vi "BatteryHPPCTest.vi"() -> ()   [LabVIEW 2020]
uses:
  <instrlib>/NH Research Regenerative Test Series/Public/Configure/Output Safety.ctl
  <instrlib>/NH Research Regenerative Test Series/NH Research Regenerative Test Series.lvlib
panel:
  out "error out":errorcluster
  out "Wait after discharge":dbl caption="Elapsed Time (s)"
  out "wait before discharge":dbl caption="Elapsed Time (s)"
  out "wait after pulse":dbl caption="Elapsed Time (s)"
  out "initial Wait":dbl caption="Elapsed Time (s)"
  in  "DAQmx Task Name":refnum<k21>
  out "String":string
  in  "5-SOC steps":T1 {"Voltage Setpoint (0 V) 3" format="%#.6g"; "Current Setpoint (0 A) 3" format="%#.6g"; "Power Setpoint (0 W) 3" format="%#.6g"; "Resistance Setpoint (0 Ohms) 3" format="%#.6g"; "Voltage Setpoint (0 V) 2" format="%#.6g"; "Current Setpoint (0 A) 2" format="%#.6g"; "Power Setpoint (0 W) 2" format="%#.6g"; "Resistance Setpoint (0 Ohms) 2" format="%#.6g"; "Voltage Setpoint (0 V)" format="%#.6g"; "Current Setpoint (0 A)" format="%#.6g"; "Power Setpoint (0 W)" format="%#.6g"; "Resistance Setpoint (0 Ohms)" format="%#.6g"; "Battery Detect Voltage (0V)" format="%#.6g"}
  in  "10-SOC steps":T2 {"Voltage Setpoint (0 V) 3" format="%#.6g"; "Current Setpoint (0 A) 3" format="%#.6g"; "Power Setpoint (0 W) 3" format="%#.6g"; "Resistance Setpoint (0 Ohms) 3" format="%#.6g"; "Voltage Setpoint (0 V) 2" format="%#.6g"; "Current Setpoint (0 A) 2" format="%#.6g"; "Power Setpoint (0 W) 2" format="%#.6g"; "Resistance Setpoint (0 Ohms) 2" format="%#.6g"; "Voltage Setpoint (0 V)" format="%#.6g"; "Current Setpoint (0 A)" format="%#.6g"; "Power Setpoint (0 W)" format="%#.6g"; "Resistance Setpoint (0 Ohms)" format="%#.6g"; "Battery Detect Voltage (0V)" format="%#.6g"}
  in  "#5-SOC steps":i32
  in  "#10-SOC Steps":i32
  in  "Output Safety":T3
  in  "VISA resource name":refnum<visa-resource-name>
  # "For Discharge Pulse:"
  # "For Charge Pulse:"
  # "For  5SOC discharge:"
  # "For Discharge Pulse:"
  # "For Charge Pulse:"
  # "For  10SOC discharge:"
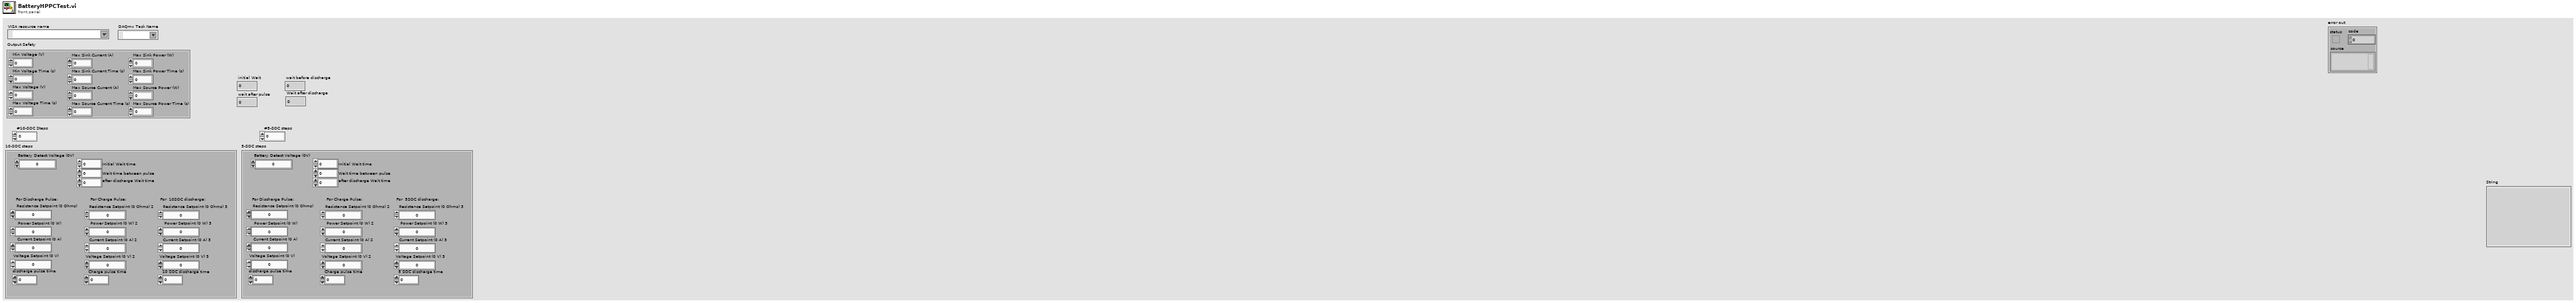
[diagram p1: front panel]
types:
  T1 = cluster{"Battery Detect Voltage (0V)":dbl, "Initial Wait time":dbl, "Resistance Setpoint (0 Ohms)":dbl, "Power Setpoint (0 W)":dbl, "Current Setpoint (0 A)":dbl, "Voltage Setpoint (0 V)":dbl, "Wait time between pulse":dbl, "after discharge Wait time ":dbl, "Resistance Setpoint (0 Ohms) 2":dbl, "Power Setpoint (0 W) 2":dbl, "Current Setpoint (0 A) 2":dbl, "Voltage Setpoint (0 V) 2":dbl, "Resistance Setpoint (0 Ohms) 3":dbl, "Power Setpoint (0 W) 3":dbl, "Current Setpoint (0 A) 3":dbl, "Voltage Setpoint (0 V) 3":dbl, "discharge pulse time":dbl, "Charge pulse time ":dbl, "5 SOC discharge time":dbl}
  T2 = cluster{"Battery Detect Voltage (0V)":dbl, "Initial Wait time":dbl, "Resistance Setpoint (0 Ohms)":dbl, "Power Setpoint (0 W)":dbl, "Current Setpoint (0 A)":dbl, "Voltage Setpoint (0 V)":dbl, "Wait time between pulse":dbl, "after discharge Wait time ":dbl, "Resistance Setpoint (0 Ohms) 2":dbl, "Power Setpoint (0 W) 2":dbl, "Current Setpoint (0 A) 2":dbl, "Voltage Setpoint (0 V) 2":dbl, "Resistance Setpoint (0 Ohms) 3":dbl, "Power Setpoint (0 W) 3":dbl, "Current Setpoint (0 A) 3":dbl, "Voltage Setpoint (0 V) 3":dbl, "discharge pulse time":dbl, "Charge pulse time ":dbl, "10 SOC discharge time":dbl}
  T3 = typedef "NH Research Regenerative Test Series.lvlib/Output Safety.ctl" = cluster{"Min Voltage (V)":dbl, "Min Voltage Time (s)":dbl, "Max Voltage (V)":dbl, "Max Voltage Time (s)":dbl, "Max Sink Current (A)":dbl, "Max Sink Current Time (s)":dbl, "Max Source Current (A)":dbl, "Max Source Current Time (s)":dbl, "Max Sink Power (W)":dbl, "Max Sink Power Time (s)":dbl, "Max Source Power (W)":dbl, "Max Source Power Time (s)":dbl}
  T4 = cluster{"[0]":refnum<visa-resource-name>, "[1]":refnum<visa-resource-name>, "[2]":refnum<visa-resource-name>, "[3]":refnum<visa-resource-name>, "[4]":refnum<visa-resource-name>, "[5]":refnum<visa-resource-name>, "[6]":refnum<visa-resource-name>, "[7]":refnum<visa-resource-name>, "[8]":refnum<visa-resource-name>}
  T5 = cluster{"[0]":refnum<k21>, "[1]":refnum<k21>, "[2]":refnum<k21>, "[3]":refnum<k21>, "[4]":refnum<k21>, "[5]":refnum<k21>, "[6]":refnum<k21>, "[7]":refnum<k21>, "[8]":refnum<k21>}
  T6 = cluster{"[0]":errorcluster, "[1]":errorcluster, "[2]":errorcluster, "[3]":errorcluster, "[4]":errorcluster, "[5]":errorcluster, "[6]":errorcluster, "[7]":errorcluster, "[8]":errorcluster}
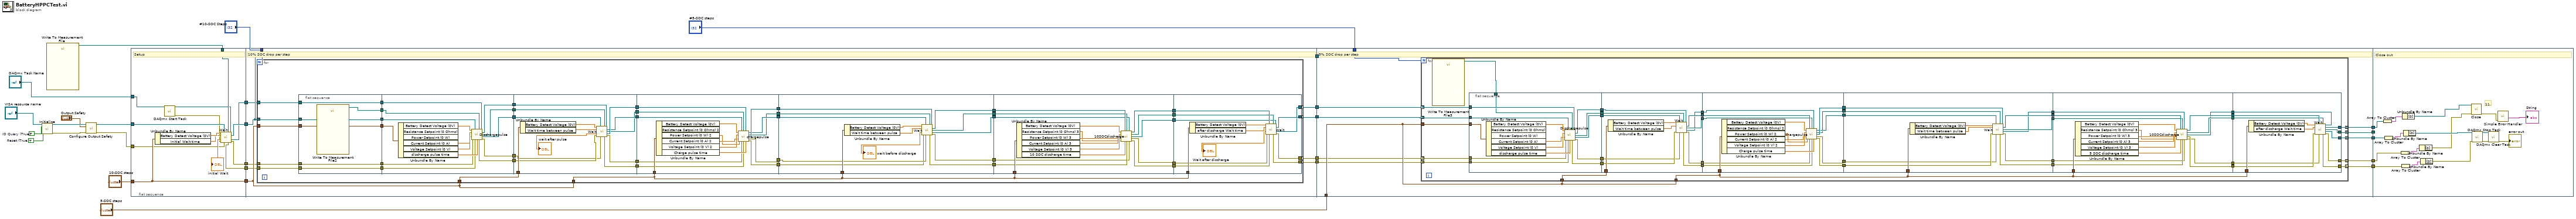
[diagram p0: block diagram]
diagram:
  w28 = TRUE  # ID Query (True)
  w27 = TRUE  # Reset (True)
  n1 = call <vilib>:"Initialize.vi"("VISA resource name"="VISA resource name", "ID Query (True)"=w28, "Reset (True)"=w27) -> ("VISA resource name out"=w26:refnum<visa-resource-name>, "error out"=w25:errorcluster)  [unwired: 11 in]
  n2 = call "Write To Measurement File"() -> ("Filename Out"=w11:path)  [unwired: 17 in, 2 out]
  n3 = call <vilib>:"Configure Output Safety.vi"("VISA resource name"=w26, "Output Safety"="Output Safety", "error in (no error)"=w25) -> ("VISA resource name out"=w23:refnum<visa-resource-name>, "error out"=w10:errorcluster)  [unwired: 11 in]
  n4 = flat-sequence {
    tunnel: w23 -> [w35]
    tunnel: [w36] -> w20
    tunnel: "10-SOC steps" -> [w43]
    tunnel: [w43] -> w17
    tunnel: "DAQmx Task Name" -> [w30]
    tunnel: [w33] -> w14
    tunnel: w11 -> [w34]
    tunnel: w10 -> [w39]
    tunnel: [w38] -> w9
    tunnel: [w37] -> w8
    tunnel: "#10-SOC Steps" -> [w53]
    tunnel: w20 -> [w50]
    tunnel: [w52] -> w19
    tunnel: w17 -> [w51]
    tunnel: [w50] -> w15
    tunnel: w14 -> [w49]
    tunnel: [w48] -> w13
    tunnel: w9 -> [w47]
    tunnel: w8 -> [w46]
    tunnel: [w45] -> w7
    tunnel: [w44] -> w6
    tunnel: "#5-SOC steps" -> [w200]
    tunnel: w19 -> [w201]
    tunnel: "5-SOC steps" -> [w199]
    tunnel: w15 -> [_]
    tunnel: w13 -> [w198]
    tunnel: w7 -> [w197]
    tunnel: w6 -> [w196]
    tunnel: [w195] -> w5
    tunnel: [w194] -> w4
    tunnel: [w193] -> w3
    tunnel: [w192] -> w2
    tunnel: [w191] -> w1
    tunnel: w5 -> [w336]
    tunnel: w4 -> [w338]
    tunnel: w3 -> [w342]
    tunnel: w2 -> [_]
    tunnel: w1 -> [w340]
    frame #0 {
      # "Setup"
      n5 = Unbundle By Name(w43) -> ("Battery Detect Voltage (0V)"=w42:dbl, "Initial Wait time"=w41:dbl)
      n6 = call <vilib>:"DAQmx Start Task.vi"("task/channels in"=w30) -> ("task out"=w31:refnum<k21>, "error out"=w32:errorcluster)  [unwired: 13 in]
      n7 = call "Wait.vi"("Battery Detect Voltage (0V)"=w42, "VISA resource name"=w35, "Path"=w34, "DAQmx Task Name"=w31, "Wait time"=w41, "Task error in"=w32, "Visa error in (no error)"=w39) -> ("VISA resource name out"=w36:refnum<visa-resource-name>, "WaitElapsed Time (s)"=→"initial Wait":dbl, "task out"=w33:refnum<k21>, "Task error out"=w37:errorcluster, "Visa error out"=w38:errorcluster)  [unwired: 3 in, 1 out]
    }
    frame #1 {
      # "10% SOC drop per step"
      n8 = for {
        N: w53 -> [_]
        tunnel: w50 -> [w91]
        tunnel: [w90] -> w52 mode=indexing
        tunnel: w51 -> [w89]
        tunnel: w51 -> [w88]
        tunnel: w51 -> [w87]
        tunnel: w49 -> [w86]
        tunnel: [w80] -> w48 mode=indexing
        tunnel: w47 -> [w79]
        tunnel: w46 -> [w78]
        tunnel: [w61] -> w45 mode=indexing
        tunnel: [w60] -> w44 mode=indexing
        n9 = flat-sequence {
          tunnel: w78 -> [w97]
          tunnel: w79 -> [w98]
          tunnel: w86 -> [w99]
          tunnel: w89 -> [w100]
          tunnel: w91 -> [w101]
          tunnel: [w101] -> w59
          tunnel: [w100] -> w58
          tunnel: [w99] -> w57
          tunnel: [w98] -> w56
          tunnel: [w97] -> w55
          tunnel: [w96] -> w54
          tunnel: [w104] -> w95
          tunnel: [w105] -> w85
          tunnel: [w109] -> w77
          tunnel: [w108] -> w76
          tunnel: [w103] -> w75
          tunnel: w59 -> [w107]
          tunnel: w58 -> [w116]
          tunnel: w57 -> [w106]
          tunnel: w56 -> [w111]
          tunnel: w55 -> [w110]
          tunnel: w54 -> [w102]
          tunnel: w95 -> [w119]
          tunnel: [w121] -> w94
          tunnel: w88 -> [w130]
          tunnel: w85 -> [w118]
          tunnel: [w122] -> w84
          tunnel: w77 -> [w126]
          tunnel: w76 -> [w125]
          tunnel: w75 -> [w117]
          tunnel: [w124] -> w74
          tunnel: [w123] -> w73
          tunnel: [w120] -> w72
          tunnel: w94 -> [w131]
          tunnel: [w135] -> w93
          tunnel: w87 -> [w146]
          tunnel: w84 -> [w132]
          tunnel: [w136] -> w83
          tunnel: w74 -> [w139]
          tunnel: w73 -> [w140]
          tunnel: w72 -> [w133]
          tunnel: [w134] -> w71
          tunnel: [w138] -> w70
          tunnel: [w137] -> w69
          tunnel: w93 -> [w156]
          tunnel: w87 -> [w160]
          tunnel: w83 -> [w154]
          tunnel: [w152] -> w82
          tunnel: w71 -> [w155]
          tunnel: w70 -> [w149]
          tunnel: w69 -> [w150]
          tunnel: [w153] -> w68
          tunnel: [w151] -> w67
          tunnel: [w148] -> w65
          tunnel: [w147] -> w64
          tunnel: [w167] -> w92
          tunnel: w87 -> [w177]
          tunnel: w82 -> [w170]
          tunnel: [w166] -> w81
          tunnel: w68 -> [w169]
          tunnel: w67 -> [w168]
          tunnel: [w165] -> w66
          tunnel: w65 -> [w164]
          tunnel: w64 -> [w163]
          tunnel: [w162] -> w63
          tunnel: [w161] -> w62
          tunnel: w92 -> [w184]
          tunnel: [w181] -> w90
          tunnel: w87 -> [w190]
          tunnel: w81 -> [w182]
          tunnel: [w180] -> w80
          tunnel: w66 -> [w183]
          tunnel: w63 -> [w185]
          tunnel: w62 -> [w186]
          tunnel: [w179] -> w61
          tunnel: [w178] -> w60
          frame #0 {
            n10 = call "Write To Measurement File2"() -> ("Filename Out"=w96:path)  [unwired: 17 in, 2 out]
          }
          frame #1 {
            n11 = Unbundle By Name(w116) -> ("Battery Detect Voltage (0V)"=w115:dbl, "Current Setpoint (0 A)"=w113:dbl, "Voltage Setpoint (0 V)"=w114:dbl, "discharge pulse time"=w112:dbl)  [unwired: 2 out]
            n12 = call "Dischargepulse.vi"("Battery Detect Voltage (0V)"=w115, "VISA resource name"=w107, "Path"=w102, "DAQmx Task Name"=w106, "Voltage Setpoint (0 V)"=w114, "Current Setpoint (0 A)"=w113, "error in (no error)"=w111, "Task error in"=w110, "pulse time"=w112) -> ("task out"=w105:refnum<k21>, "Filename Out"=w103:path, "VISA resource name out"=w104:refnum<visa-resource-name>, "Task error out 2"=w109:errorcluster, "error out"=w108:errorcluster)  [unwired: 2 in]
          }
          frame #2 {
            n13 = Unbundle By Name(w130) -> ("Battery Detect Voltage (0V)"=w129:dbl, "Wait time between pulse"=w128:dbl)
            n14 = call "Wait.vi"("Battery Detect Voltage (0V)"=w129, "VISA resource name"=w119, "Path"=w117, "DAQmx Task Name"=w118, "Wait time"=w128, "Task error in"=w126, "Visa error in (no error)"=w125) -> ("VISA resource name out"=w121:refnum<visa-resource-name>, "Filename Out"=w120:path, "WaitElapsed Time (s)"=→"wait after pulse":dbl, "task out"=w122:refnum<k21>, "Task error out"=w124:errorcluster, "Visa error out"=w123:errorcluster)  [unwired: 3 in]
          }
          frame #3 {
            n15 = Unbundle By Name(w146) -> ("Battery Detect Voltage (0V)"=w145:dbl, "Power Setpoint (0 W) 2"=w142:dbl, "Current Setpoint (0 A) 2"=w143:dbl, "Voltage Setpoint (0 V) 2"=w144:dbl, "Charge pulse time"=w141:dbl)  [unwired: 1 out]
            n16 = call "chargepulse.vi"("Battery Detect Voltage (0V)"=w145, "VISA resource name"=w131, "Path"=w133, "DAQmx Task Name"=w132, "Voltage Setpoint (0 V)"=w144, "Current Setpoint (0 A)"=w143, "Power Setpoint (0 W)"=w142, "error in (no error)"=w140, "Task error in"=w139, "pulse time"=w141) -> ("VISA resource name out"=w135:refnum<visa-resource-name>, "Filename Out"=w134:path, "task out"=w136:refnum<k21>, "error out"=w137:errorcluster, "Task error out"=w138:errorcluster)  [unwired: 1 in]
          }
          frame #4 {
            n17 = Unbundle By Name(w160) -> ("Battery Detect Voltage (0V)"=w159:dbl, "Wait time between pulse"=w158:dbl)
            n18 = call "Wait.vi"("Battery Detect Voltage (0V)"=w159, "VISA resource name"=w156, "Path"=w155, "DAQmx Task Name"=w154, "Wait time"=w158, "Task error in"=w149, "Visa error in (no error)"=w150) -> ("VISA resource name out"=w152:refnum<visa-resource-name>, "Filename Out"=w151:path, "WaitElapsed Time (s)"=→"wait before discharge":dbl, "task out"=w153:refnum<k21>, "Task error out"=w148:errorcluster, "Visa error out"=w147:errorcluster)  [unwired: 3 in]
          }
          frame #5 {
            n19 = Unbundle By Name(w177) -> ("Battery Detect Voltage (0V)"=w176:dbl, "Resistance Setpoint (0 Ohms) 3"=w172:dbl, "Power Setpoint (0 W) 3"=w173:dbl, "Current Setpoint (0 A) 3"=w174:dbl, "Voltage Setpoint (0 V) 3"=w175:dbl, "10 SOC discharge time"=w171:dbl)
            n20 = call "10SOCdischarge.vi"("Battery Detect Voltage (0V)"=w176, "VISA resource name"=w170, "Path"=w168, "DAQmx Task Name"=w169, "Voltage Setpoint (0 V)"=w175, "Current Setpoint (0 A)"=w174, "Power Setpoint (0 W)"=w173, "Resistance Setpoint (0 Ohms)"=w172, "Discharge time"=w171, "Task error in"=w164, "error in (no error)"=w163) -> ("VISA resource name out"=w167:refnum<visa-resource-name>, "Filename Out"=w165:path, "task out"=w166:refnum<k21>, "Task error out 2"=w161:errorcluster, "error out"=w162:errorcluster)
          }
          frame #6 {
            n21 = Unbundle By Name(w190) -> ("Battery Detect Voltage (0V)"=w189:dbl, "after discharge Wait time"=w188:dbl)
            n22 = call "Wait.vi"("Battery Detect Voltage (0V)"=w189, "VISA resource name"=w184, "Path"=w183, "DAQmx Task Name"=w182, "Wait time"=w188, "Task error in"=w186, "Visa error in (no error)"=w185) -> ("VISA resource name out"=w181:refnum<visa-resource-name>, "WaitElapsed Time (s)"=→"Wait after discharge":dbl, "task out"=w180:refnum<k21>, "Task error out"=w179:errorcluster, "Visa error out"=w178:errorcluster)  [unwired: 3 in, 1 out]
          }
        }
      }
    }
    frame #2 {
      # "5% SOC drop per step"
      n23 = for {
        N: w200 -> [_]
        tunnel: w201 -> [w234] mode=indexing
        tunnel: w199 -> [w233]
        tunnel: w199 -> [w232]
        tunnel: w199 -> [w231]
        tunnel: w198 -> [w230] mode=indexing
        tunnel: w197 -> [w223] mode=indexing
        tunnel: w196 -> [w222] mode=indexing
        tunnel: [w206] -> w195 mode=indexing
        tunnel: [w205] -> w194 mode=indexing
        tunnel: [w204] -> w193 mode=indexing
        tunnel: [w203] -> w192 mode=indexing
        tunnel: [w202] -> w191 mode=indexing
        n24 = call "Write To Measurement File3"() -> ("Filename Out"=w224:path)  [unwired: 17 in, 2 out]
        n25 = flat-sequence {
          tunnel: w224 -> [w243]
          tunnel: [w241] -> w239
          tunnel: w234 -> [w245]
          tunnel: w233 -> [w254]
          tunnel: w230 -> [w244]
          tunnel: [w242] -> w229
          tunnel: w223 -> [w248]
          tunnel: w222 -> [w249]
          tunnel: [w247] -> w221
          tunnel: [w246] -> w220
          tunnel: [w240] -> w219
          tunnel: w239 -> [w264]
          tunnel: [w257] -> w238
          tunnel: w232 -> [w267]
          tunnel: w229 -> [w263]
          tunnel: [w255] -> w228
          tunnel: w221 -> [w261]
          tunnel: w220 -> [w260]
          tunnel: w219 -> [w262]
          tunnel: [w259] -> w218
          tunnel: [w258] -> w217
          tunnel: [w256] -> w216
          tunnel: w238 -> [w281]
          tunnel: [w269] -> w237
          tunnel: w231 -> [w283]
          tunnel: w228 -> [w282]
          tunnel: [w270] -> w227
          tunnel: w218 -> [w273]
          tunnel: w217 -> [w274]
          tunnel: w216 -> [w280]
          tunnel: [w272] -> w215
          tunnel: [w271] -> w214
          tunnel: [w268] -> w213
          tunnel: w237 -> [w286]
          tunnel: [w289] -> w236
          tunnel: w231 -> [w296]
          tunnel: w227 -> [w284]
          tunnel: [w287] -> w226
          tunnel: w215 -> [w293]
          tunnel: w214 -> [w292]
          tunnel: w213 -> [w285]
          tunnel: [w291] -> w212
          tunnel: [w290] -> w211
          tunnel: [w288] -> w210
          tunnel: w236 -> [w312]
          tunnel: [w299] -> w235
          tunnel: w231 -> [w313]
          tunnel: w226 -> [w311]
          tunnel: [w297] -> w225
          tunnel: w212 -> [w303]
          tunnel: w211 -> [w302]
          tunnel: w210 -> [w310]
          tunnel: [w301] -> w209
          tunnel: [w300] -> w208
          tunnel: [w298] -> w207
          tunnel: w235 -> [w315]
          tunnel: w231 -> [w326]
          tunnel: w225 -> [w316]
          tunnel: w209 -> [w323]
          tunnel: w208 -> [w322]
          tunnel: w207 -> [w314]
          tunnel: [w321] -> w206
          tunnel: [w320] -> w205
          tunnel: [w319] -> w204
          tunnel: [w318] -> w203
          tunnel: [w317] -> w202
          frame #0 {
            n26 = Unbundle By Name(w254) -> ("Battery Detect Voltage (0V)"=w253:dbl, "Current Setpoint (0 A)"=w251:dbl, "Voltage Setpoint (0 V)"=w252:dbl, "discharge pulse time"=w250:dbl)  [unwired: 2 out]
            n27 = call "Dischargepulse.vi"("Battery Detect Voltage (0V)"=w253, "VISA resource name"=w245, "Path"=w243, "DAQmx Task Name"=w244, "Voltage Setpoint (0 V)"=w252, "Current Setpoint (0 A)"=w251, "error in (no error)"=w249, "Task error in"=w248, "pulse time"=w250) -> ("task out"=w242:refnum<k21>, "Filename Out"=w240:path, "VISA resource name out"=w241:refnum<visa-resource-name>, "Task error out 2"=w247:errorcluster, "error out"=w246:errorcluster)  [unwired: 2 in]
          }
          frame #1 {
            n28 = Unbundle By Name(w267) -> ("Battery Detect Voltage (0V)"=w266:dbl, "Wait time between pulse"=w265:dbl)
            n29 = call "Wait.vi"("Battery Detect Voltage (0V)"=w266, "VISA resource name"=w264, "Path"=w262, "DAQmx Task Name"=w263, "Wait time"=w265, "Task error in"=w261, "Visa error in (no error)"=w260) -> ("VISA resource name out"=w257:refnum<visa-resource-name>, "Filename Out"=w256:path, "task out"=w255:refnum<k21>, "Task error out"=w259:errorcluster, "Visa error out"=w258:errorcluster)  [unwired: 3 in, 1 out]
          }
          frame #2 {
            n30 = Unbundle By Name(w283) -> ("Battery Detect Voltage (0V)"=w279:dbl, "Power Setpoint (0 W) 2"=w276:dbl, "Current Setpoint (0 A) 2"=w277:dbl, "Voltage Setpoint (0 V) 2"=w278:dbl, "Charge pulse time"=w275:dbl)  [unwired: 1 out]
            n31 = call "chargepulse.vi"("Battery Detect Voltage (0V)"=w279, "VISA resource name"=w281, "Path"=w280, "DAQmx Task Name"=w282, "Voltage Setpoint (0 V)"=w278, "Current Setpoint (0 A)"=w277, "Power Setpoint (0 W)"=w276, "error in (no error)"=w274, "Task error in"=w273, "pulse time"=w275) -> ("VISA resource name out"=w269:refnum<visa-resource-name>, "Filename Out"=w268:path, "task out"=w270:refnum<k21>, "error out"=w271:errorcluster, "Task error out"=w272:errorcluster)  [unwired: 1 in]
          }
          frame #3 {
            n32 = Unbundle By Name(w296) -> ("Battery Detect Voltage (0V)"=w295:dbl, "Wait time between pulse"=w294:dbl)
            n33 = call "Wait.vi"("Battery Detect Voltage (0V)"=w295, "VISA resource name"=w286, "Path"=w285, "DAQmx Task Name"=w284, "Wait time"=w294, "Task error in"=w293, "Visa error in (no error)"=w292) -> ("VISA resource name out"=w289:refnum<visa-resource-name>, "Filename Out"=w288:path, "task out"=w287:refnum<k21>, "Task error out"=w291:errorcluster, "Visa error out"=w290:errorcluster)  [unwired: 3 in, 1 out]
          }
          frame #4 {
            n34 = Unbundle By Name(w313) -> ("Battery Detect Voltage (0V)"=w309:dbl, "Resistance Setpoint (0 Ohms) 3"=w305:dbl, "Power Setpoint (0 W) 3"=w306:dbl, "Current Setpoint (0 A) 3"=w307:dbl, "Voltage Setpoint (0 V) 3"=w308:dbl, "5 SOC discharge time"=w304:dbl)
            n35 = call "10SOCdischarge.vi"("Battery Detect Voltage (0V)"=w309, "VISA resource name"=w312, "Path"=w310, "DAQmx Task Name"=w311, "Voltage Setpoint (0 V)"=w308, "Current Setpoint (0 A)"=w307, "Power Setpoint (0 W)"=w306, "Resistance Setpoint (0 Ohms)"=w305, "Discharge time"=w304, "Task error in"=w303, "error in (no error)"=w302) -> ("VISA resource name out"=w299:refnum<visa-resource-name>, "Filename Out"=w298:path, "task out"=w297:refnum<k21>, "Task error out 2"=w301:errorcluster, "error out"=w300:errorcluster)
          }
          frame #5 {
            n36 = Unbundle By Name(w326) -> ("Battery Detect Voltage (0V)"=w325:dbl, "after discharge Wait time"=w324:dbl)
            n37 = call "Wait.vi"("Battery Detect Voltage (0V)"=w325, "VISA resource name"=w315, "Path"=w314, "DAQmx Task Name"=w316, "Wait time"=w324, "Task error in"=w323, "Visa error in (no error)"=w322) -> ("VISA resource name out"=w319:refnum<visa-resource-name>, "Filename Out"=w318:path, "task out"=w317:refnum<k21>, "Task error out"=w321:errorcluster, "Visa error out"=w320:errorcluster)  [unwired: 3 in, 1 out]
          }
        }
      }
    }
    frame #3 {
      # "11."
      # "Close out"
      n38 = Array To Cluster(array=w342) -> (cluster=w328:T4)
      n39 = Array To Cluster(array=w340) -> (cluster=w341:T5)
      n40 = Array To Cluster(array=w338) -> (cluster=w339:T6)
      n41 = Array To Cluster(array=w336) -> (cluster=w337:T6)
      n42 = Unbundle By Name(w328) -> ("[0]"=w327:refnum<visa-resource-name>)
      n43 = Unbundle By Name(w341) -> ("[0]"=w335:refnum<k21>)
      n44 = Unbundle By Name(w339) -> ("[0]"=w330:errorcluster)
      n45 = Unbundle By Name(w337) -> ("[0]"=w334:errorcluster)
      n46 = call <instrlib>:"Close.vi"("VISA resource name"=w327, "error in (no error)"=w330) -> ("error out"=w329:errorcluster)  [unwired: 13 in]
      n47 = call <vilib>:"DAQmx Stop Task.vi"("task/channels in"=w335, "error in"=w334) -> ("task out"=w333:refnum<k21>, "error out"=w332:errorcluster)  [unwired: 12 in]
      n48 = call <vilib>:"DAQmx Clear Task.vi"("task in"=w333, "error in"=w332) -> ("error out"=→"error out":errorcluster)  [unwired: 13 in]
      n49 = call <vilib>:"Simple Error Handler.vi"("error in (no error)"=w329) -> ("source out"=→"String":string)  [unwired: 4 in, 4 out]
    }
  }
